vi "ExQCircBuf.vi"() -> ()   [LabVIEW 2010]
uses:
  Open-Close/CamHandle.vi
panel:
  in  "Exposure":dbl min=0.0 step=0.001 format="%.3f"
  in  "stop":bool
  in  "Store":bool
  out "error out":errorcluster
  in  "error in (no error)":errorcluster
  # "ExQCircBuf:\nThis example allows a full image\nto be programmed up. It then runs\nin sync (focus) mode displaying \nthe full image data as it comes in.\nNote: this example requires the \ncamera support circular buffers."
  # "NOTICE\n\nTHIS VI USES A GLOBAL CAMERA HANDLE\n\nTHE VI EXOPENGLOBALCAM.VI MUST BE\nRUN AT THE START OF THE WORK SESSION.\nTHE CAMERA WILL REMAIN OPENED.\n\nTHE VI EXCLOSEGLOBALCAM.VI MUST\nBE RUN BEFORE LEAVING LABVIEW."
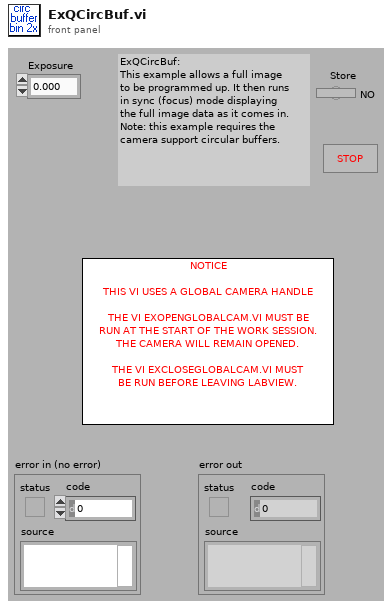
[diagram p1: front panel]
types:
  T1 = cluster{"acquire focus mode":u32, "Exposure":dbl, "Number of Images":u32, "Software accumulation":u32}
  T2 = cluster{"Camera Handle":u32, "File Handle":u32, "Display Handle":u32, "Image Handle":u32}
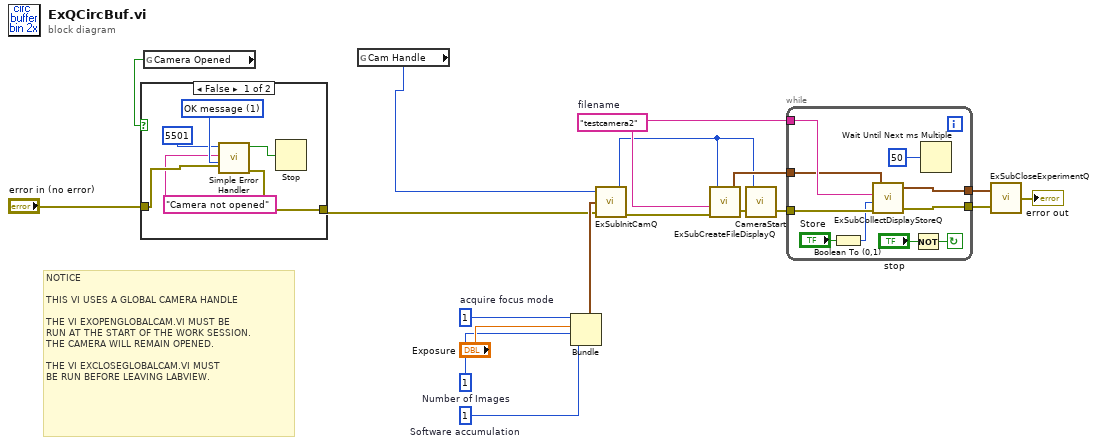
[diagram p0: block diagram]
diagram:
  w8 = u32 1  # acquire focus mode
  w7 = u32 1  # Number of Images
  w6 = u32 1  # Software accumulation
  w18 = "testcamera2"  # filename
  # "NOTICE\n\nTHIS VI USES A GLOBAL CAMERA HANDLE\n\nTHE VI EXOPENGLOBALCAM.VI MUST BE\nRUN AT THE START OF THE WORK SESSION.\nTHE CAMERA WILL REMAIN OPENED.\n\nTHE VI EXCLOSEGLOBALCAM.VI MUST\nBE RUN BEFORE LEAVING LABVIEW."
  n1 = global read "CamHandle.vi" "Camera Opened"() -> (w3:bool)
  n2 = case shown="False" w3 {
    tunnel: "error in (no error)" -> [w23 w25]
    tunnel: [w22 w25] -> w1
    frame False {
      w24 = u16 1 items=["no dialog", "OK message", "continue or stop message"] ("type of dialog (OK msg:1)")
      n3 = call <vilib>:"Simple Error Handler.vi"("error code (no error:0)"=5501, "error source (\" \")"="Camera not opened", "type of dialog (OK msg:1)"=w24, "error in (no error)"=w23) -> ("error?"=w20:bool, "error out"=w22:errorcluster)  [unwired: 1 in, 3 out]
      n4 = Stop(stop? (T)=w20) -> ()
    }
    frame True {
    }
  }
  n5 = global read "CamHandle.vi" "Cam Handle"() -> (w2:u32)
  n6 = Bundle("acquire focus mode"=w8, "Exposure"="Exposure", "Number of Images"=w7, "Software accumulation"=w6) -> (w16:T1)  [unwired: 1 in]
  n7 = call "ExSubInitCamQ.vi"("error in (no error)"=w1, "Camera Information"=w16, "Camera Handle"=w2) -> ("error out"=w15:errorcluster, "Camera Handle"=w5:u32)
  n8 = call "ExSubCreateFileDisplayQ.vi"("error in (no error)"=w15, "File and Display Name"=w18, "Camera Handle"=w5) -> ("error out"=w9:errorcluster, "Handles Out"=w14:T2)  [unwired: 1 in]
  n9 = call <userlib>:"CameraStart.vi"("error in"=w9, "Camera Handle"=w5) -> ("error out"=w10:errorcluster)  [unwired: 1 out]
  n10 = while {
    tunnel: w14 -> [w26]
    tunnel: w10 -> [w34]
    tunnel: w18 -> [w27]
    tunnel: [w32] -> w12
    tunnel: [w33] -> w13
    stop <- w30 continue-if-true
    n11 = Boolean To (0,1)(Boolean="Store") -> (0, 1=w28:i16)
    n12 = call "ExSubCollectDisplayStoreQ.vi"("error in (no error)"=w34, "Store flag"=w28, "Display Title"=w27, "Handle Cluster"=w26) -> ("error out"=w32:errorcluster, "Handle Cluster Out"=w33:T2)  [unwired: 1 out]
    n13 = Not(x="stop") -> (.not. x?=w30:bool)
    n14 = Wait Until Next ms Multiple(millisecond multiple=u32 50) -> ()  [unwired: 1 out]
  }
  n15 = call "ExSubCloseExperimentQ.vi"("error in (no error)"=w12, "Handles In"=w13) -> ("error out"=→"error out":errorcluster)
